vi "Waveform - Min Max.vi"() -> ()   [LabVIEW 2023]
doc: "Shows how to use the Waveform Min Max VI to extract the maximum and minimum from a waveform."
panel:
  out "Waveform Graph":waveform(dbl)(graph)
  out "Minimum Time":timestamp
  out "Maximum Time":timestamp
  out "Minimum Value":dbl format="%.2f"
  out "Maximum Value":dbl format="%.2f"
  # "Overview: Demonstrates how to acquire information about the minimum and maximum values in a waveform with the Waveform Min Max VI.\nInstructions:\nRun the VI. The minimum and maximum values within the waveform are displayed, along with timestamps specifying when those values occurred."
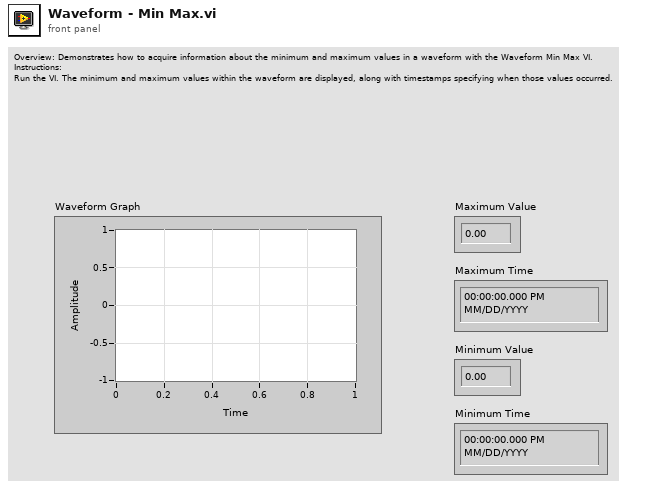
[diagram p1: front panel]
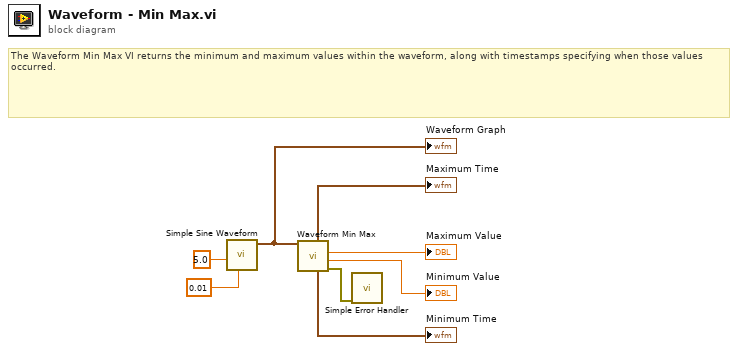
[diagram p0: block diagram]
diagram:
  # "The Waveform Min Max VI returns the minimum and maximum values within the waveform, along with timestamps specifying when those values occurred."
  n1 = call "Simple Sine Waveform.vi"("delta t"=0.01, "n cycles"=5.0 ("frequency")) -> ("sine waveform"=w1:waveform(dbl))  [unwired: 9 in]
  "Waveform Graph" <- w1
  n2 = call <vilib>:"Waveform Min Max.vi"("waveform in"=w1) -> ("error out"=w2:errorcluster, "Y min"=→"Minimum Value":dbl, "Y max"=→"Maximum Value":dbl, "min time"=→"Minimum Time":timestamp, "max time"=→"Maximum Time":timestamp)  [unwired: 5 in, 1 out]
  n3 = call <vilib>:"Simple Error Handler.vi"("error in (no error)"=w2) -> ()  [unwired: 4 in, 5 out]
